vi "init_vi_calcul.vi"() -> ()   [LabVIEW 2025]
panel:
  out "Frequency":dbl format="%#_3p"
  in  "C":dbl
  in  "L":dbl
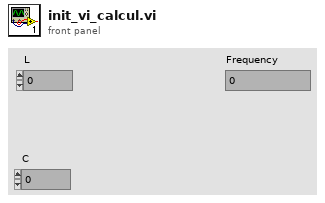
[diagram p1: front panel]
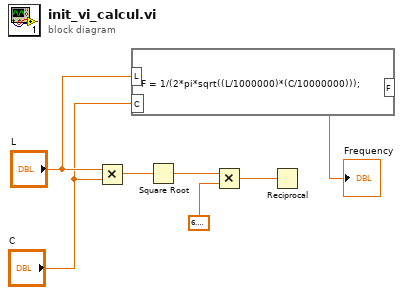
[diagram p0: block diagram]
diagram:
  n1 = Multiply(x="L", y="C") -> (x*y=w6:dbl)
  n2 = formula code="F = 1/(2*pi*sqrt((L/1000000)*(C/10000000)));"("L"="L", "C"="C") -> ("F"=→"Frequency":dbl)
  n3 = Square Root(x=w6) -> (sqrt(x)=w7:dbl)
  n4 = Multiply(x=w7, y=6.283185307179586) -> (x*y=w5:dbl)
  n5 = Reciprocal(x=w5) -> ()  [unwired: 1 out]
